vi "Safety Xor by Array.vi"(8 "error in (no error)":errorcluster, 10 "Digital In":bool[](array[boolean]), 11 "DIG_IO in":refnum<class "DIG_IO.lvclass">) -> (0 "error out":errorcluster, 2 "Digital Out":bool[](array[boolean]), 3 "DIG_IO out":refnum<class "DIG_IO.lvclass">)   [LabVIEW 2019, in "DIG_IO.lvlib" / "DIG_IO.lvclass"]
uses:
  Library/DIG_IO.lvclass
  Library/DIG_IO.lvclass/DIG_IO.ctl
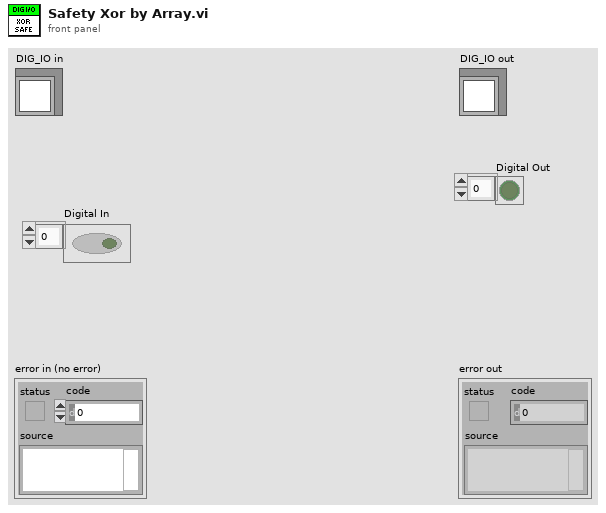
[diagram p1: front panel]
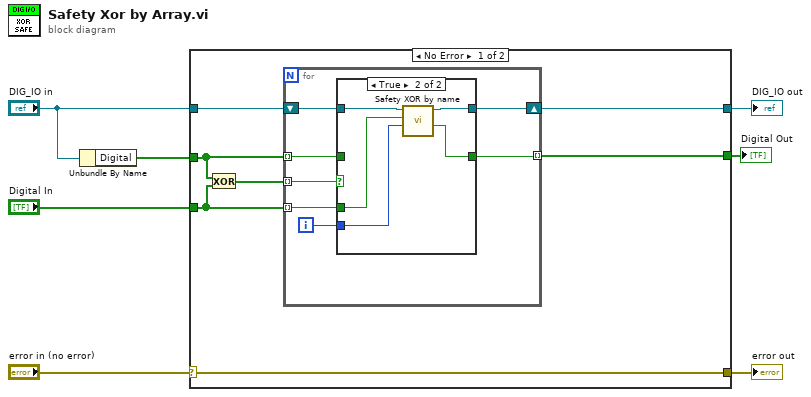
[diagram p0: block diagram]
diagram:
  n1 = Unbundle By Name("DIG_IO in") -> ("Digital"=w2:bool[])
  n2 = case shown="No Error" "error in (no error)" {
    selector: "error in (no error)" -> [w14 w30]
    tunnel: [w14 w30] -> w6
    tunnel: [w9 w29] -> w5
    tunnel: "DIG_IO in" -> [w10 w29]
    tunnel: "Digital In" -> [w12 _]
    tunnel: w2 -> [w11 _]
    tunnel: [w8 _] -> w1
    frame No Error {
      n3 = Exclusive Or(1:w12, 2:w11) -> (0:w13:bool[])
      n4 = for {
        tunnel: w13 -> [w21] mode=indexing
        tunnel: w12 -> [w20] mode=indexing
        tunnel: w11 -> [w18] mode=indexing
        tunnel: [w17] -> w8 mode=indexing
        shift-right: [w15] -> w9
        shift-left: w10 -> [w16]
        i -> [w19]
        n5 = case shown="True" w21 {
          tunnel: w20 -> [_ w24]
          tunnel: w19 -> [_ w28]
          tunnel: w18 -> [w23 _]
          tunnel: [w23 w25] -> w17
          tunnel: w16 -> [w22 w27]
          tunnel: [w22 w26] -> w15
          frame False {
          }
          frame True {
            n6 = call "Safety XOR by name.vi"("Target Digital in"=w28, "Value to Write"=w24, "DIG_IO in"=w27) -> ("Value Select"=w25:bool, "DIG_IO out"=w26:refnum<class "DIG_IO.lvclass">)  [unwired: 5 in, 2 out]
          }
        }
      }
    }
    frame Error {
    }
  }
  "error out" <- w6
  "DIG_IO out" <- w5
  "Digital Out" <- w1
